vi "Set channel parameters.vi"(8 "error in (no error)":errorcluster, 11 "Channel Req in":refnum<class "Channel Req.lvclass">) -> (0 "error out":errorcluster, 3 "Channel Req out":refnum<class "Channel Req.lvclass">)   [LabVIEW 2018, in "Channel Req.lvclass"]
uses:
  Channel Req.lvclass
  <vilib>/addons/zeromq/socket_type.ctl
  Socket2/Socket2/Socket2.lvclass
  <vilib>/addons/zeromq/zeromq.lvlib
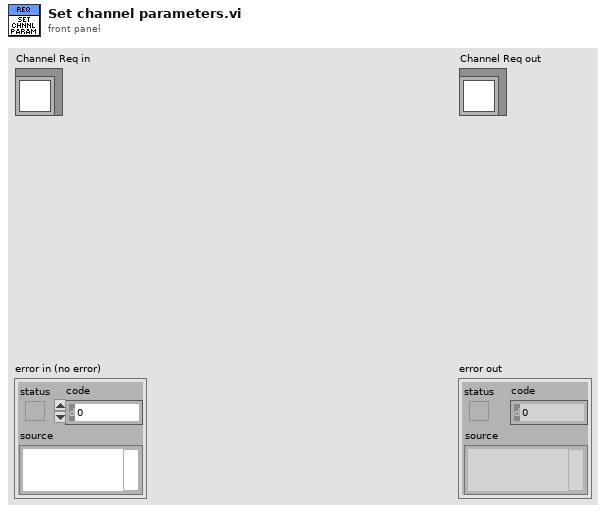
[diagram p1: front panel]
types:
  T1 = typedef "zeromq.lvlib/socket_type.ctl" = enum8{"ZMQ_PAIR", "ZMQ_PUB", "ZMQ_SUB", "ZMQ_REQ", "ZMQ_REP", "ZMQ_DEALER", "ZMQ_ROUTER", "ZMQ_PULL", "ZMQ_PUSH", "ZMQ_XPUB", "ZMQ_XSUB", "ZMQ_STREAM", "ZMQ_SERVER", "ZMQ_CLIENT", "ZMQ_RADIO", "ZMQ_DISH", "ZMQ_GATHER", "ZMQ_SCATTER", "ZMQ_DGRAM"}
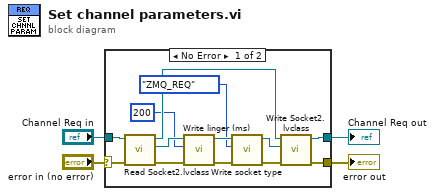
[diagram p0: block diagram]
diagram:
  n1 = case shown="No Error" "error in (no error)" {
    selector: "error in (no error)" -> [w7 w18]
    tunnel: "Channel Req in" -> [w8 w19]
    tunnel: [w6 w19] -> w2
    tunnel: [w5 w18] -> w1
    frame No Error {
      n2 = call-dynamic "Read Socket2.lvclass.vi"("error in (no error)"=w7, "Communication Channel in"=w8) -> ("error out"=w11:errorcluster, "Socket2.lvclass"=w16:refnum<class "Socket2.lvclass">, "Communication Channel out"=w17:refnum<class "Channel Req.lvclass">)  [unwired: 7 in]
      n3 = call-dynamic "Write linger (ms).vi"("error in (no error)"=w11, "linger (ms)"=200, "Socket in"=w16) -> ("error out"=w12:errorcluster, "Socket out"=w15:refnum<class "Socket2.lvclass">)  [unwired: 7 in]
      n4 = call-dynamic "Write socket type.vi"("error in (no error)"=w12, "Socket type"=socket_type."ZMQ_REQ", "Socket in"=w15) -> ("error out"=w13:errorcluster, "Socket out"=w14:refnum<class "Socket2.lvclass">)  [unwired: 7 in]
      n5 = call-dynamic "Write Socket2.lvclass.vi"("error in (no error)"=w13, "Socket2.lvclass"=w14, "Communication Channel in"=w17) -> ("error out"=w5:errorcluster, "Communication Channel out"=w6:refnum<class "Channel Req.lvclass">)  [unwired: 7 in]
    }
    frame Error {
    }
  }
  "error out" <- w1
  "Channel Req out" <- w2
